vi "Timestamp_Convert Difference to dt Increments.vi"(7 "Dt":dbl=1.0, 10 "Start Time":timestamp, 11 "End Time":timestamp) -> (2 "Round Up Dt Increment Out":i32, 3 "Nearest Dt Increment Out":i32, 5 "Round Down Dt Increment Out":i32)   [LabVIEW 2024]
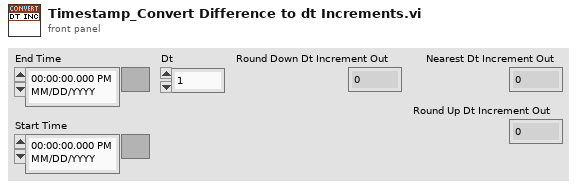
[diagram p1: front panel]
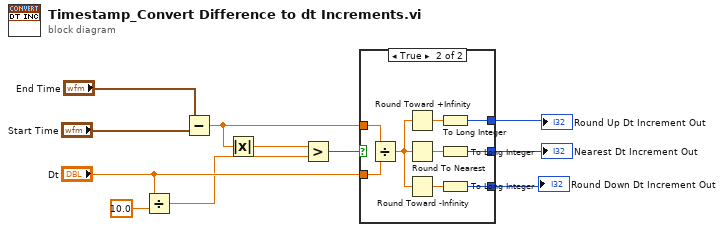
[diagram p0: block diagram]
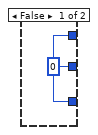
[diagram p2: hidden frame]
diagram:
  n1 = Divide(x="Dt", y=10.0) -> (x/y=w2:dbl)
  n2 = Subtract(x="End Time", y="Start Time") -> (x-y=w8:dbl)
  n3 = Absolute Value(x=w8) -> (abs(x)=w1:dbl)
  n4 = Greater?(x=w1, y=w2) -> (0:w7:bool)
  n5 = case shown="True" w7 {
    tunnel: [w12 w21] -> w11
    tunnel: "Dt" -> [_ w20]
    tunnel: w8 -> [_ w18]
    tunnel: [w12 w16] -> w6
    tunnel: [w12 w13] -> w5
    frame False {
      w12 = 0
    }
    frame True {
      n6 = Divide(x=w18, y=w20) -> (x/y=w15:dbl)
      n7 = Round Toward +Infinity(x=w15) -> (ceil(x): smallest int >= x=w17:dbl)
      n8 = Round To Nearest(number=w15) -> (nearest integer value=w19:dbl)
      n9 = Round Toward -Infinity(1:w15) -> (0:w14:dbl)
      n10 = To Long Integer(number=w17) -> (32bit integer=w16:i32)
      n11 = To Long Integer(number=w19) -> (32bit integer=w21:i32)
      n12 = To Long Integer(number=w14) -> (32bit integer=w13:i32)
    }
  }
  "Nearest Dt Increment Out" <- w11
  "Round Up Dt Increment Out" <- w6
  "Round Down Dt Increment Out" <- w5
